vi "Robot Global Data.vi"() -> ()   [LabVIEW 2017]
doc: "This global VI can contain as many global variables as you need. To create a global variable, place a control on the panel, give it a good name. To read or write to it from a VI, drag the icon to the diagram of that VI. You can also drag from the project. Click on the node to change which global you access. You shouldn't have multiple locations writing to a global or it will cause a race-condition."
uses:
  <vilib>/Rock Robotics/WPI/Camera/WPI_CameraImageSize.ctl
  <vilib>/Rock Robotics/WPI/DriverStation/WPI_DriverStationRobotMode2.ctl
  <vilib>/Rock Robotics/WPI/DriverStation/WPI_DriverStationPositionInfo.ctl
panel:
  in  "Hook Arm Up Setpoint":dbl=1.0
  in  "Hook Arm Down Setpoint":dbl=-1.0
  in  "Climber Setpoint":dbl
  in  "Climber Time (ms)":dbl
  in  "Climber Button":bool
  in  "Hook Up Setpoint":dbl
  in  "Hook Down Setpoint":dbl
  in  "Select Data Source":enum16{"auto.csv", "Robot Main"}(ring)
  out "Autonomous Data Robot Main":string[][](array[string])=[["", "Left Speed", "Right Speed", "Time", "Left Speed", "Right Speed", "Time", "Left Speed", "Right Speed", "Time", "Left Speed", "Right Speed", "Time", "Left Speed", "Right Speed", "Time"], ["Robot Left Switch Left", "-0.5", "-0.5", "4000", "-0.5", "0.5", "1000", "-0.5", "-0.5", "2000", "", "", "", "", "", ""], ["Robot Right Switch Right", "-0.5", "-0.5", "4000", "0.5", "-0.5", "1000", "-0.5", "-0.5", "2000", "", "", "", "", "", ""], ["Robot Left Switch Right", "-1", "-1", "3000", "-0.5", "0.5", "1000", "-1", "-1", "5000", "-0.5", "0.5", "1000", "-0.5", "-0.5", "2000"], ["Robot Right Switch Left", "-1", "-1", "3000", "0.5", "-0.5", "1000", "-1", "-1", "5000", "0.5", "-0.5", "1000", "-0.5", "-0.5", "2000"], ["Robot Middle Switch Left", "-1", "-1", "724", "", "", "", "", "", "", "", "", "", "", "", ""], ["Robot Middle Switch Right", "-1", "-1", "724", "", "", "", "", "", "", "", "", "", "", "", ""]]
  in  "Auto by Time Raise Arm Time (ms)":dbl=1000.0
  in  "Auto by Time Lower Cube Time (ms)":dbl=1000.0
  in  "Auto by Time Release CubeTime (ms)":dbl=1000.0
  in  "Robot Position Selector":T1(ring)=enum."Robot Position for Debug"
  in  "Auto type":enum16{"Auto by Time", "Auto by Loops"}(ring)
  in  "Switch Position for debugging":string="R"
  in  "Robot Position for debugging":T2=enum."2"
  in  "Auto by Loops Raise Arm Time (ms)":dbl
  in  "Auto by Loops Lower Cube Time (ms)":dbl
  in  "Auto by Loops Release CubeTime (ms)":dbl
  in  "Switch Position":string="R"
  in  "Robot Position":T2=enum."2"
  out "Autonomous Data":T3(array[cluster])
  in  "Hook UpTime (ms)":dbl
  in  "Hook DownTime (ms)":dbl
  in  "Move Hook Down Button":bool
  in  "Move Hook Up Button":bool
  in  "Backwards Button":bool
  in  "Forward Button":bool
  in  "Backward Time (ms)":dbl
  in  "Forward Time (ms)":dbl
  in  "Hook Arm UpTime (ms)":dbl
  in  "Hook Arm DownTime (ms)":dbl
  in  "Move Hook Arm Down Button":bool
  in  "Move Hook Arm Up Button":bool
  in  "Clear PDP Sticky Fault":bool
  in  "Move Hook Arm":dbl
  in  "Move Hook":dbl
  in  "Move Grabber":dbl
  in  "Move Arm":dbl
  in  "Right Turn Button":bool
  in  "Left Turn Button":bool
  in  "Drive Turn":dbl
  in  "Drive Speed":dbl
  in  "Right Turn Time (ms)":dbl
  in  "Left Turn Time (ms)":dbl
  in  "Rate reduction":dbl
  in  "Min Output(0 to 1)":dbl
  in  "Select Mode":T4(ring)=enum."Exponential"
  in  "n^x(Unbounded)":dbl=2.5 format="%#_13g"
  in  "Sonar Distance":dbl
  in  "Robot Mode":T5
  in  "image size":T6=enum."320x240"
  in  "Enable Vision":bool
  # "Drive Settings"
  # "Hook Settings"
  # "Climber Settings"
  # "Auto Settings"
  # "Joystick 0 Values"
  # "Joystick 1 Values"
  # "Autonomous Settings"
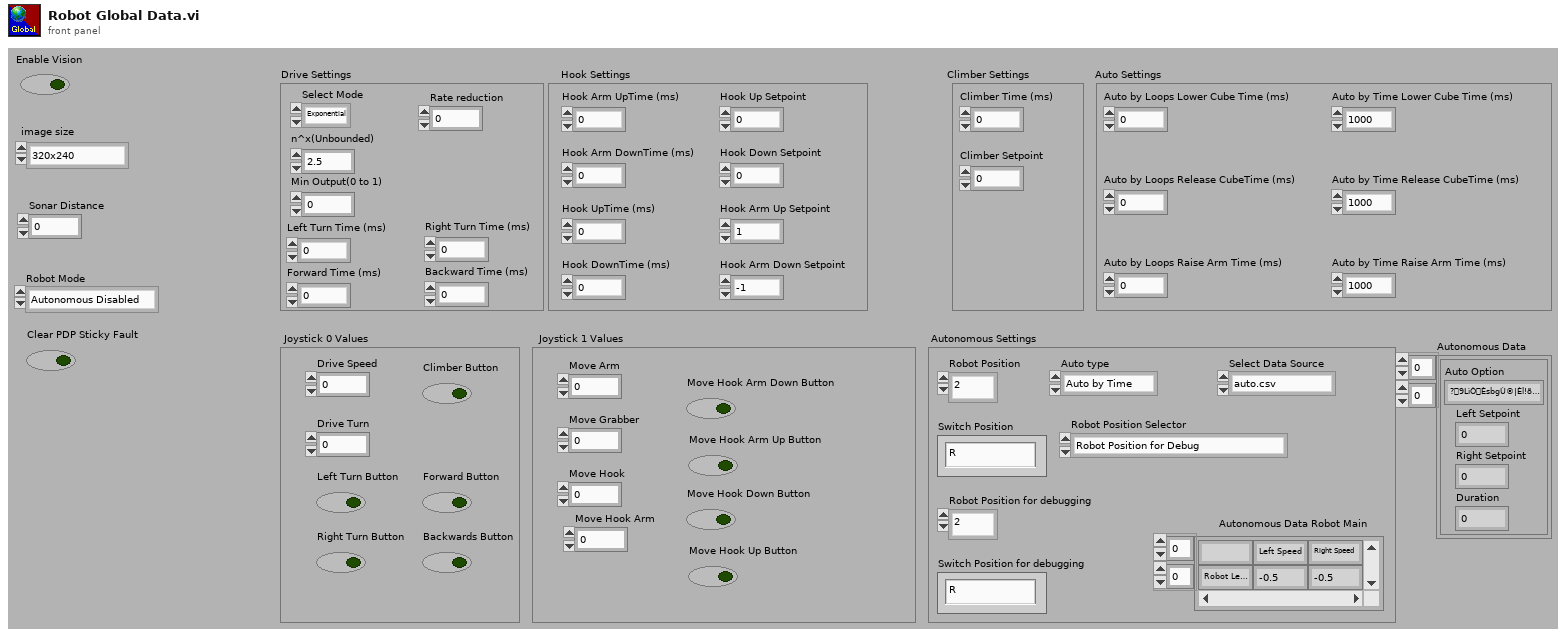
[diagram p1: front panel]
types:
  T1 = enum16{"Robot Position from the FMS", "Robot Position from the Dashboard", "Robot Position for Debug"}
  T2 = typedef "WPI_DriverStationPositionInfo.ctl" = enum16{"1", "2", "3"}
  T3 = cluster{"Auto Option":string, "Left Setpoint":dbl, "Right Setpoint":dbl, "Duration":dbl}[][]
  T4 = enum16{"Normal", "Square", "Square with Rate", "Square Root", "Linear", "Exponential"}
  T5 = typedef "WPI_DriverStationRobotMode2.ctl" = enum16{"Autonomous Disabled", "Autonomous Enabled", "Teleop Disabled", "Teleop Enabled", "Disconnected", "Finish", "Test Disabled", "Test Enabled", "Emergency Stopped"}
  T6 = typedef "WPI_CameraImageSize.ctl" = enum16{"640x480", "320x240", "160x120", "Custom"}
diagram:
